vi "ToplevelMicroZedSerialController.vi"() -> ()   [LabVIEW 2014]
uses:
  c_MicroZedInstr_Enum.ctl
  g_MicroZed_Interface.vi
panel:
  in  "COM Port MicroZed":refnum<visa-resource-name>="COM4"
  in  "Parameters":string
  in  "Run Timer":bool
  out "Test Timeout":bool
  out "Busy":bool
  out "Terminal":string
  out "read buffer":string
  in  "Start":bool
  in  "Command":T1
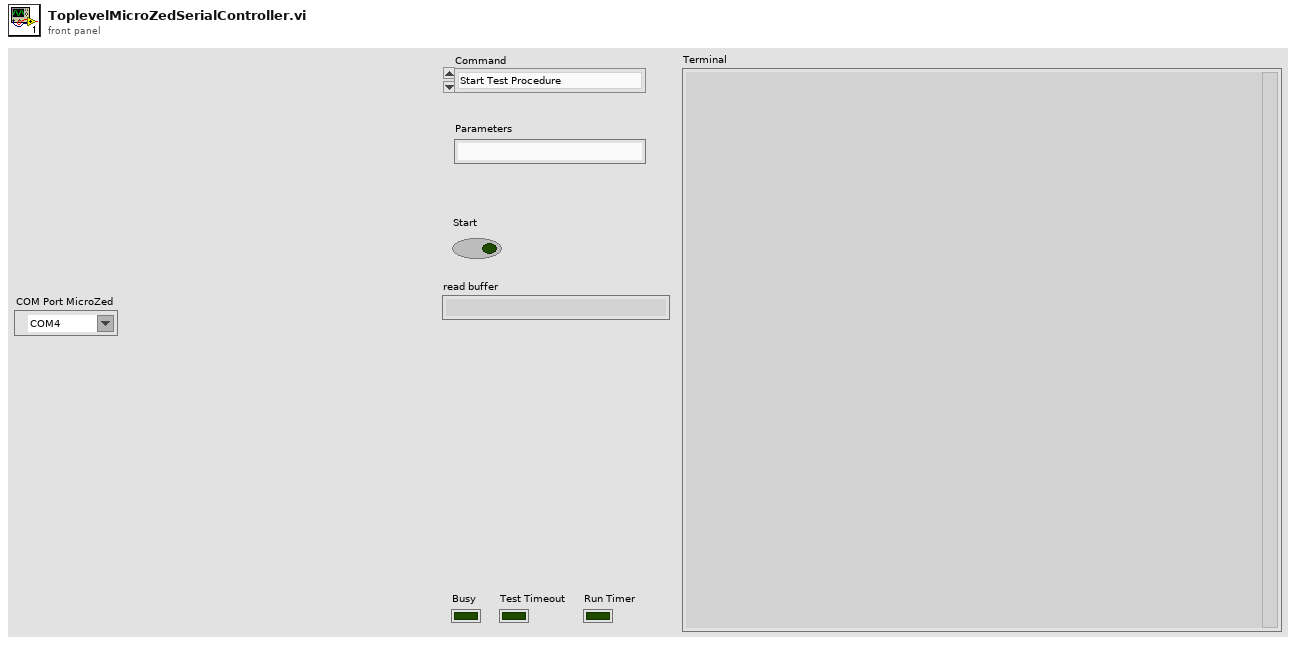
[diagram p1: front panel]
types:
  T1 = typedef "c_MicroZedInstr_Enum.ctl" = enum16{"Start Test Procedure", "Print Instructions", "Config HCC Register", "Send Parameters"}
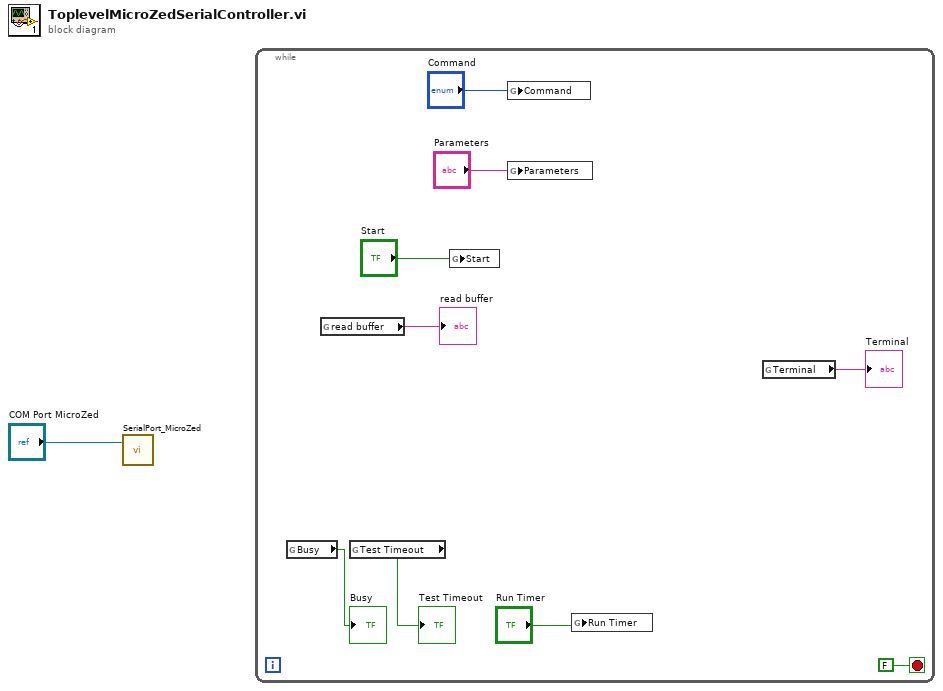
[diagram p0: block diagram]
diagram:
  n1 = call "SerialPort_MicroZed.vi"("COM Port"="COM Port MicroZed") -> ()  [unwired: 2 in, 1 out]
  n2 = while {
    stop <- FALSE stop-if-true
    n3 = global read "g_MicroZed_Interface.vi" "Busy"() -> (→"Busy":bool)
    n4 = global read "g_MicroZed_Interface.vi" "read buffer"() -> (→"read buffer":string)
    n5 = global read "g_MicroZed_Interface.vi" "Test Timeout"() -> (→"Test Timeout":bool)
    n6 = global write "g_MicroZed_Interface.vi" "Start"("Start") -> ()
    n7 = global write "g_MicroZed_Interface.vi" "Command"("Command") -> ()
    n8 = global write "g_MicroZed_Interface.vi" "Parameters"("Parameters") -> ()
    n9 = global write "g_MicroZed_Interface.vi" "Run Timer"("Run Timer") -> ()
    n10 = global read "g_MicroZed_Interface.vi" "Terminal"() -> (→"Terminal":string)
  }
